vi "Save.vi"() -> ()   [LabVIEW 2016]
uses:
  Set Save Object Dictionary.vi
  <vilib>/CANopenLib/CANOPEN.llb/CANopen SDO Create.vi
  <vilib>/CANopenLib/CANOPEN.llb/CANopen SDO Write.vi
  <vilib>/CANopenLib/CANOPEN.llb/CANopen SDO Write [STR].vi
  <vilib>/CANopenLib/CANOPEN.llb/CANopen SDO Close.vi
panel:
  out "completion code":u32
  in  "Motor":u8(ring) items=["Right", "Left"]
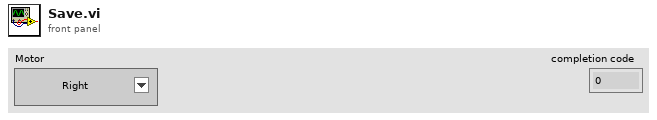
[diagram p1: front panel]
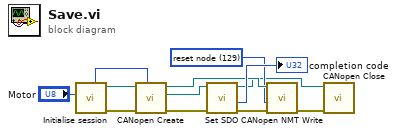
[diagram p0: block diagram]
diagram:
  w4 = u16 129 items=["start remote node"=1, "stop remote node"=2, "enter pre-operational"=128, "reset node"=129, "reset communication"=130] ("command")
  n1 = call "Initialise session.vi"("Motor"="Motor") -> ("error out"=w12:errorcluster, "interface object out"=w11:refnum<k20>, "Used Node ID"=w8:u8)  [unwired: 8 in]
  n2 = call-poly <vilib>:"CANopen Create.vi"("node-ID"=w8, "error in (no error)"=w12, "interface object in"=w11) -> ("error out"=w10:errorcluster, "SDO object out"=w9:refnum<k20>, "interface object out"=w5:refnum<k20>)  [unwired: 6 in]
  n3 = call-poly "Set SDO.vi"("error in (no error)"=w10, "SDO object in"=w9) -> ("error out"=w3:errorcluster, "completion code"=→"completion code":u32, "SDO object out"=w1:refnum<k20>)  [unwired: 7 in]
  n4 = call <vilib>:"CANopen NMT Write.vi"("error in (no error)"=w3, "command"=w4, "interface object in"=w5) -> ("error out"=w2:errorcluster)  [unwired: 7 in, 1 out]
  n5 = call-poly <vilib>:"CANopen Close.vi"("error in (no error)"=w2, "SDO object in"=w1) -> ()  [unwired: 9 in, 1 out]
